vi "PDE Thermal Distribution.vi"() -> ()   [LabVIEW 2023]
doc: "This example demonstrates how to use the Partial Differential Equations VIs to define and solve a 2-dimensional heat equation on rectangular domain. Suppose that there is a thin square plate. Two boundaries of the plate lose heat to the surrounding with fixed rate. On the other two boundaries the temperatures are not varied. At initial time, the temperatures in the plate are all zero. If there is an external source to heat the plate, the temperatures start changing. As time evolves, the thermal distribution approaches an equilibrium state. The 2-dimensional heat equation in this example describes the thermal distribution in the thin square plate over time."
uses:
  <vilib>/gmath/pde.llb/Common/PDE_BC Type.ctl
  <vilib>/gmath/pde.llb/Common/PDE_BC Position 2D.ctl
  <vilib>/Analysis/1siggen.llb/Ramp Pattern by Samples.vi
  <vilib>/gmath/pde.llb/Define 2D Heat PDE (VIRef).vi
  <vilib>/gmath/pde.llb/Define 2D Heat PDE Domain (Rect).vi
  <vilib>/gmath/pde.llb/Define 2D Heat PDE BC (VIRef).vi
  <vilib>/gmath/pde.llb/Define 2D Heat PDE IC (Numeric).vi
  <vilib>/gmath/pde.llb/2D Heat PDE Solver (Rect Domain).vi
  <vilib>/gmath/pde.llb/2D Heat PDE Rendering (Rect Domain).vi
  <vilib>/gmath/NI_PDE.lvlib
  <vilib>/Analysis/NI_AALBase.lvlib
panel:
  out "End Y":T1(graph)
  out "End X":T1(graph)
  out "Start Y":T1(graph)
  out "Start X":T1(graph)
  out "Solution":dbl[][](graph)
  out "Heat Source":dbl[][](graph)
  out "Current Time (s)":dbl(slide) scale=0.0..5.0
  in  "Temperature":i32(slide)=50 scale=0.0..100.0
  in  "Y Range":dbl(slide)=0.010205858847733066 scale=0.001..0.1 scale format="%#.3g"
  in  "X Range":dbl(slide)=0.010205858847733066 scale=0.001..0.1 scale format="%#.3g"
  in  "Y Center":dbl(slide)=0.496969696969697 scale=0.2..0.8 scale format="%#_2g"
  in  "X Center":dbl(slide)=0.496969696969697 scale=0.2..0.8 scale format="%#_2g"
  in  "Stop":bool
  # "Overview: This example demonstrates how to use the Partial Differential Equations VIs to define and solve a 2-dimensional heat equation in a rectangular domain.\nRequirements: LabVIEW Full Development System\nInstructions: \n1. Change the various Heat Source Parameters.\n2. Run the VI to see the thermal distribution in the thin square plate.\n3. Click Stop to stop the VI.\n4. Change the Heat Source Parameters and run the VI again."
  # "Temperature and Thermal Flux on Boundaries"
  # "Heat Source Parameters"
  # "Temperature"
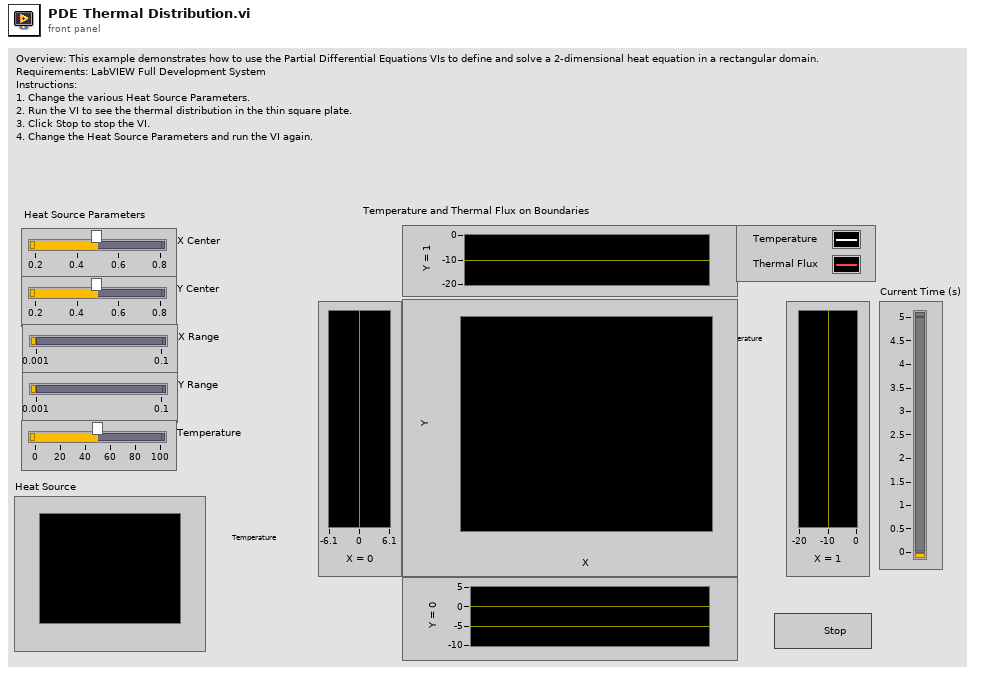
[diagram p1: front panel]
types:
  T1 = cluster{"Ramp Pattern":dbl[], "U(t, x, y)":dbl[]}[]
  T2 = cluster{"initial t":dbl, "final t":dbl, "# of t-points":i32}
  T3 = cluster{"start x":dbl, "end x":dbl, "# of x-points":i32}
  T4 = typedef "NI_PDE.lvlib/PDE_BC Position 2D.ctl" = i32
  T5 = typedef "NI_PDE.lvlib/PDE_BC Type.ctl" = i32
  T6 = cluster{"Temperature":i32, "X Center":dbl, "Y Center":dbl, "X Range":dbl, "Y Range":dbl}
  T7 = typedef "LVOffsetAndMultiplierTypeDef.ctl" = cluster{"Offset":dbl, "Multiplier":dbl}
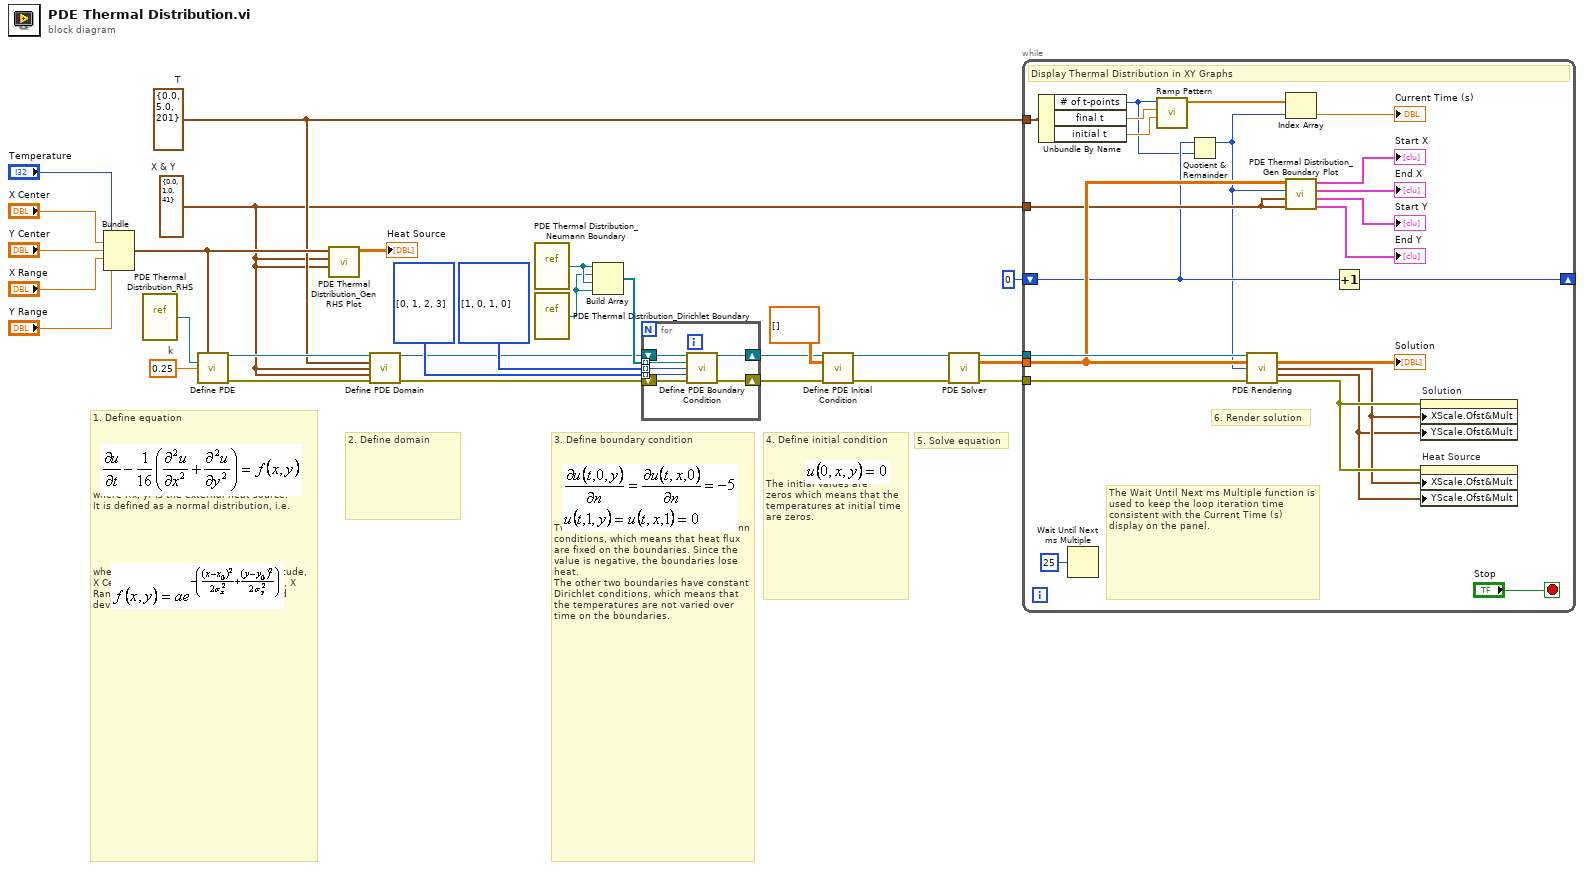
[diagram p0: block diagram]
diagram:
  w3 = T2 {"initial t"=0.0, "final t"=5.0, "# of t-points"=201}  # T
  w2 = T3 {"start x"=0.0, "end x"=1.0, "# of x-points"=41}  # X & Y
  w26 = T4[] [0, 1, 2, 3] items=["Start X", "End X", "Start Y", "End Y"]
  w27 = T5[] [1, 0, 1, 0] items=["Dirichlet", "Neumann"]
  w18 = 0.25  # k
  # "3. Define boundary condition            \n\n\n\n\n\n\n\nTwo boundaries have constant Neumann conditions, which means that heat flux are fixed on the boundaries. Since the value is negative, the boundaries lose heat.\nThe other two boundaries have constant Dirichlet conditions, which means that the temperatures are not varied over time on the boundaries."
  # "4. Define initial condition\n\n\n\nThe initial values are \nzeros which means that the temperatures at initial time are zeros."
  # "2. Define domain"
  # "5. Solve equation"
  # "1. Define equation                                     \n\n\n\n\n\n\nwhere f(x, y) is the external heat source.\nIt is defined as a normal distribution, i.e.\n\n\n\n\n\nwhere Temperature specifies the amplitude, X Center and Y Center specify the mean, X Range and Y Range specify the standard deviation of the normal distribution."
  n1 = Bundle("Temperature"="Temperature", "X Center"="X Center", "Y Center"="Y Center", "X Range"="X Range", "Y Range"="Y Range") -> (w13:T6)  [unwired: 1 out]
  n2 = vi-ref "PDE Thermal Distribution_RHS.vi"() -> (w28:refnum<vi>)
  n3 = call-poly <vilib>:"Define PDE.vi"("data"=w13, "F(t, x, y)"=w28, "k"=w18) -> ("PDE out"=w14:refnum<class "NI_PDE.lvclass">, "error out"=w17:errorcluster)  [unwired: 3 in, 8 out]
  n4 = call "PDE Thermal Distribution_Gen RHS Plot.vi"("Y"=w2, "X"=w2, "RHS Para"=w13) -> ("RHS"=→"Heat Source":dbl[][])  [unwired: 8 out]
  n5 = call-poly <vilib>:"Define PDE Domain.vi"("PDE in"=w14, "T"=w3, "X"=w2, "Y"=w2, "error in (no error)"=w17) -> ("PDE out"=w15:refnum<class "NI_PDE.lvclass">, "error out"=w16:errorcluster)  [unwired: 9 out]
  n6 = vi-ref "PDE Thermal Distribution_Neumann Boundary.vi"() -> (w24:refnum<vi>)
  n7 = vi-ref "PDE Thermal Distribution_Dirichlet Boundary.vi"() -> (w23:refnum<vi>)
  n8 = Build Array(w24, w23, w24, w23) -> (w25:refnum<vi>[])
  n9 = for {
    shift-right: [w34] -> w21
    shift-left: w15 -> [w36]
    shift-right: [w33] -> w22
    shift-left: w16 -> [w35]
    tunnel: w25 -> [w32] mode=indexing
    tunnel: w26 -> [w31] mode=indexing
    tunnel: w27 -> [w30] mode=indexing
    n10 = call-poly <vilib>:"Define PDE Boundary Condition.vi"("PDE in"=w36, "Boundary Condition"=w32, "type"=w30, "position"=w31, "error in (no error)"=w35) -> ("PDE out"=w34:refnum<class "NI_PDE.lvclass">, "error out"=w33:errorcluster)  [unwired: 1 in, 8 out]
  }
  n11 = call-poly <vilib>:"Define PDE Initial Condition.vi"("PDE in"=w21, "Initial Condition"=dbl[][] [], "error in (no error)"=w22) -> ("PDE out"=w19:refnum<class "NI_PDE.lvclass">, "error out"=w20:errorcluster)  [unwired: 1 in, 10 out]
  n12 = call-poly <vilib>:"PDE Solver.vi"("PDE in"=w19, "error in (no error)"=w20) -> ("PDE out"=w12:refnum<class "NI_PDE.lvclass">, "U(t, x, y)"=w11:dbl[][][], "error out"=w4:errorcluster)  [unwired: 11 out]
  n13 = while {
    shift-right: [w39] -> _
    shift-left: 0 -> [w40]
    tunnel: w4 -> [w43]
    tunnel: w3 -> [w42]
    tunnel: w2 -> [w41]
    tunnel: w12 -> [w45]
    tunnel: w11 -> [w44]
    stop <- "Stop" stop-if-true
    # "The Wait Until Next ms Multiple function is used to keep the loop iteration time consistent with the Current Time (s) display on the panel."
    # "6. Render solution"
    # "Display Thermal Distribution in XY Graphs"
    n14 = Unbundle By Name(w42) -> ("# of t-points"=w38:i32, "final t"=w50:dbl, "initial t"=w51:dbl)
    n15 = Wait Until Next ms Multiple(millisecond multiple=u32 25 ("milliseconds to wait")) -> ()  [unwired: 1 out]
    n16 = call-poly <vilib>:"Ramp Pattern.vi"("start"=w51, "end"=w50, "samples"=w38) -> ("Ramp Pattern"=w49:dbl[])  [unwired: 7 in, 1 out]
    n17 = Quotient & Remainder(x=w40, y=w38) -> (x-y*floor(x/y)=w37:i32)  [unwired: 1 out]
    n18 = call-poly <vilib>:"PDE Rendering.vi"("PDE in"=w45, "U(t, x, y)"=w44, "index (time step)"=w37, "error in (no error)"=w43) -> ("PDE Plot"=→"Solution":dbl[][], "X Scale"=w53:T7, "Y Scale"=w52:T7, "error out"=w54:errorcluster)  [unwired: 8 out]
    n19 = Index Array(array=w49, index=w37) -> (element=→"Current Time (s)":dbl)
    n20 = call "PDE Thermal Distribution_Gen Boundary Plot.vi"("Y"=w41, "X"=w41, "index (time step)"=w37, "U(t, x, y)"=w44) -> ("End Y"=→"End Y":T1, "Start Y"=→"Start Y":T1, "End X"=→"End X":T1, "Start X"=→"Start X":T1)  [unwired: 4 out]
    n21 = Increment(x=w40) -> (x+1=w39:i32)
    n22 = property on="Solution" class="IntGraph (strict)"(error in=w54, "XScale.Ofst&Mult"=w53, "YScale.Ofst&Mult"=w52) -> ()  [unwired: 1 in, 2 out]
    n23 = property on="Heat Source" class="IntGraph (strict)"(error in=w54, "XScale.Ofst&Mult"=w53, "YScale.Ofst&Mult"=w52) -> ()  [unwired: 1 in, 2 out]
  }
